vi "Set_Settings_Item.vi"(8 "error in (no error)":errorcluster, 10 "data":T1, 11 "IB_Settings_Item in":refnum<class "IB_Settings_Item.lvclass">) -> (0 "error out":errorcluster, 3 "IB_Settings_Item out":refnum<class "IB_Settings_Item.lvclass">)   [LabVIEW 2020, in "IB_Settings_Item.lvclass"]
uses:
  <vilib>/AppBuilder/IB_Classes/Settings_Item/IB_Settings_Item.lvclass
  <vilib>/AppBuilder/IB_Classes/Settings_Item/IB_Settings_Item.lvclass/IB_Settings_Item.ctl
  <vilib>/AppBuilder/IB_Classes/Settings_Item/IB_Settings_Item.ctl
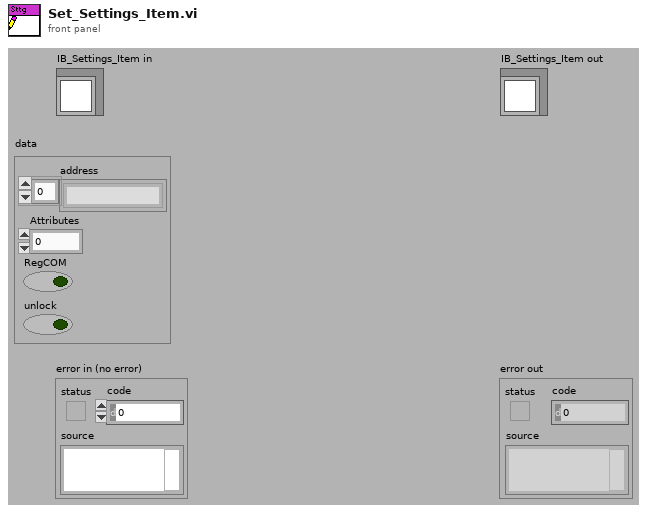
[diagram p1: front panel]
types:
  T1 = typedef "IB_Settings_Item.ctl" = cluster{"address":string[], "Attributes":i16, "RegCOM":bool, "unlock":bool}
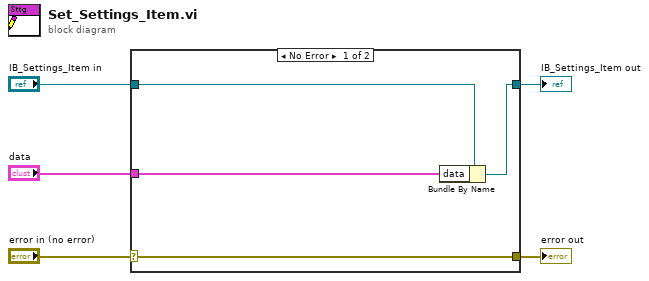
[diagram p0: block diagram]
diagram:
  n1 = case shown="No Error" "error in (no error)" {
    selector: "error in (no error)" -> [w9 w10]
    tunnel: [w9 w10] -> w4
    tunnel: [w7 w11] -> w2
    tunnel: "IB_Settings_Item in" -> [w8 w11]
    tunnel: "data" -> [w6 _]
    frame No Error {
      n2 = Bundle By Name(cluster=w8, "data"=w6) -> (w7:refnum<class "IB_Settings_Item.lvclass">)
    }
    frame Error {
    }
  }
  "error out" <- w4
  "IB_Settings_Item out" <- w2
